vi "GetInstance.vi"(7 "Logger Name (Logger)":string="Logger", 8 "error in (no error)":errorcluster) -> (0 "error out":errorcluster, 3 "RQMHLogger Get":refnum<class "RQMHLogger.lvclass">)   [LabVIEW 2024, in "RQMHLogSingleton.lvlib"]
uses:
  RQMHLogSingleton.lvlib
  RQMHLogger/RQMHLogger.lvclass
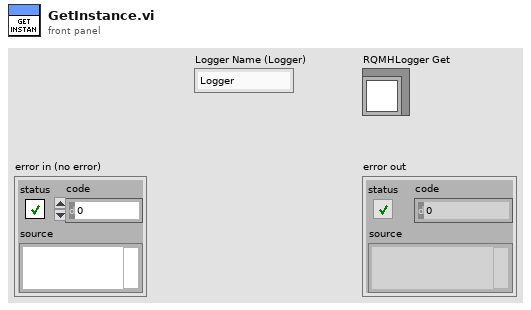
[diagram p1: front panel]
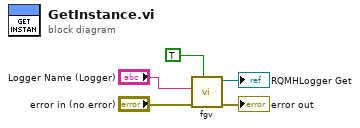
[diagram p0: block diagram]
diagram:
  n1 = call "fgv.vi"("Get? (T)"=TRUE, "error in (no error)"="error in (no error)", "Logger Name"="Logger Name (Logger)") -> ("error out"=→"error out":errorcluster, "RQMHLogger Get"=→"RQMHLogger Get":refnum<class "RQMHLogger.lvclass">)  [unwired: 7 in]
